vi "Lab Panel V4.87.vi"() -> ()   [LabVIEW 2013] (continued)
                        n2189 = case shown="True" w4030 {
                          tunnel: w4037 -> [_ w4069]
                          tunnel: w4036 -> [_ w4076]
                          tunnel: w4035 -> [_ _]
                          tunnel: w4034 -> [_ _]
                          tunnel: w4033 -> [_ w4075]
                          tunnel: w4032 -> [_ w4074]
                          tunnel: w4031 -> [_ w4039]
                          tunnel: w4028 -> [_ w4071]
                          tunnel: w4027 -> [_ w4070]
                          tunnel: w4026 -> [_ w4068]
                          tunnel: w4025 -> [_ w4060]
                          frame False {
                          }
                          frame True {
                            n2190 = local read "TDMS LAB03-1"() -> (w4073:refnum<k34>)
                            n2191 = Build Array(w4070) -> (w4065:dbl[])
                            n2192 = Build Array(w4068) -> (w4064:dbl[])
                            n2193 = Build Array(w4075) -> (w4063:dbl[])
                            n2194 = Build Array(w4076) -> (w4062:dbl[])
                            n2195 = Build Array(w4071) -> (w4067:dbl[])
                            n2196 = Build Array(w4069) -> (w4066:dbl[])
                            n2197 = Build Array(w4074) -> (w4061:dbl[])
                            n2198 = Build Array("AMPS ON", "AMPS OFF", "VOLTS", "PF", "TEMP Live", "TEMP Neut", "CYCLE") -> (w4044:string[])
                            n2199 = Bundle By Name("Y"=w4067, "t0"=w4060) -> (w4059:waveform(dbl))  [unwired: 1 in]
                            n2200 = Bundle By Name("Y"=w4066, "t0"=w4060) -> (w4058:waveform(dbl))  [unwired: 1 in]
                            n2201 = Bundle By Name("Y"=w4065, "t0"=w4060) -> (w4057:waveform(dbl))  [unwired: 1 in]
                            n2202 = Bundle By Name("Y"=w4064, "t0"=w4060) -> (w4056:waveform(dbl))  [unwired: 1 in]
                            n2203 = Bundle By Name("Y"=w4063, "t0"=w4060) -> (w4055:waveform(dbl))  [unwired: 1 in]
                            n2204 = Bundle By Name("Y"=w4062, "t0"=w4060) -> (w4054:waveform(dbl))  [unwired: 1 in]
                            n2205 = Bundle By Name("Y"=w4061, "t0"=w4060) -> (w4053:waveform(dbl))  [unwired: 1 in]
                            n2206 = Build Array(w4059, w4058, w4057, w4056, w4055, w4054, w4053) -> (w4052:waveform(dbl)[])
                            n2207 = TDMS Write(0:w4073, 5:"TEST VALUES", 7:w4044, 9:w4052) -> (4:w4043:refnum<k34>, 6:w4042:string, 15:w4041:errorcluster)  [unwired: 2 in, 1 out]
                            n2208 = TDMS Write(0:w4043, 5:w4042, 7:"TIME", 9:w4039, 11:w4041) -> (15:w4038:errorcluster)  [unwired: 1 in, 3 out]
                            n2209 = local write "data file error"(w4038) -> ()
                          }
                        }
                      }
                    }
                  }
                }
              }
              frame #5 {
                n2210 = case shown="True" w4077 {
                  tunnel: w4081 -> [_ w4086]
                  tunnel: w4080 -> [_ w4085]
                  tunnel: w4079 -> [_ w4083]
                  tunnel: w4078 -> [_ w4082]
                  frame False {
                  }
                  frame True {
                    n2211 = local read "DISP LAB03-2"() -> (w4087:T4)
                    n2212 = local read "SIG LAB03-2"() -> (w4088:T2)
                    n2213 = local read "ON L03-2"() -> (w4084:cluster{"amps":dbl, "volts":dbl, "pf":dbl})
                    n2214 = Unbundle(w4088) -> ("AMPS"=w4094:dbl, "VOLTS"=w4092:dbl, "PF"=w4091:dbl, "Tmp Live"=w4090:dbl, "Tmp Neut"=w4093:dbl)
                    n2215 = Unbundle(w4087) -> ("CYCLE"=w4089:dbl)  [unwired: 2 out]
                    n2216 = stacked-sequence {
                      tunnel: w4094 -> [w4098 w4117]
                      tunnel: w4093 -> [_ w4116]
                      tunnel: w4092 -> [w4097 w4115]
                      tunnel: w4091 -> [w4096 w4114]
                      tunnel: w4090 -> [_ w4113]
                      tunnel: w4089 -> [_ w4112]
                      tunnel: w4086 -> [_ w4111]
                      tunnel: w4085 -> [w4099 _]
                      tunnel: w4084 -> [w4095 w4109]
                      tunnel: w4083 -> [_ w4110]
                      tunnel: w4082 -> [_ w4105]
                      frame #0 {
                        n2217 = case shown="True" w4099 {
                          tunnel: w4098 -> [_ w4104]
                          tunnel: w4097 -> [_ w4103]
                          tunnel: w4096 -> [_ w4102]
                          tunnel: w4095 -> [_ w4100]
                          frame False {
                          }
                          frame True {
                            n2218 = Bundle(cluster=w4100, "amps"=w4104, "volts"=w4103, "pf"=w4102) -> (w4101:cluster{"amps":dbl, "volts":dbl, "pf":dbl})
                            n2219 = local write "ON L03-2"(w4101) -> ()
                          }
                        }
                      }
                      frame #1 {
                        n2220 = Unbundle(w4109) -> ("amps"=w4108:dbl, "volts"=w4107:dbl, "pf"=w4106:dbl)
                        n2221 = case shown="True" w4110 {
                          tunnel: w4117 -> [_ w4149]
                          tunnel: w4116 -> [_ w4156]
                          tunnel: w4115 -> [_ _]
                          tunnel: w4114 -> [_ _]
                          tunnel: w4113 -> [_ w4155]
                          tunnel: w4112 -> [_ w4154]
                          tunnel: w4111 -> [_ w4119]
                          tunnel: w4108 -> [_ w4151]
                          tunnel: w4107 -> [_ w4150]
                          tunnel: w4106 -> [_ w4148]
                          tunnel: w4105 -> [_ w4140]
                          frame False {
                          }
                          frame True {
                            n2222 = local read "TDMS LAB03-2"() -> (w4153:refnum<k34>)
                            n2223 = Build Array(w4150) -> (w4145:dbl[])
                            n2224 = Build Array(w4148) -> (w4144:dbl[])
                            n2225 = Build Array(w4155) -> (w4143:dbl[])
                            n2226 = Build Array(w4156) -> (w4142:dbl[])
                            n2227 = Build Array(w4151) -> (w4147:dbl[])
                            n2228 = Build Array(w4149) -> (w4146:dbl[])
                            n2229 = Build Array(w4154) -> (w4141:dbl[])
                            n2230 = Build Array("AMPS ON", "AMPS OFF", "VOLTS", "PF", "TEMP Live", "TEMP Neut", "CYCLE") -> (w4124:string[])
                            n2231 = Bundle By Name("Y"=w4147, "t0"=w4140) -> (w4139:waveform(dbl))  [unwired: 1 in]
                            n2232 = Bundle By Name("Y"=w4146, "t0"=w4140) -> (w4138:waveform(dbl))  [unwired: 1 in]
                            n2233 = Bundle By Name("Y"=w4145, "t0"=w4140) -> (w4137:waveform(dbl))  [unwired: 1 in]
                            n2234 = Bundle By Name("Y"=w4144, "t0"=w4140) -> (w4136:waveform(dbl))  [unwired: 1 in]
                            n2235 = Bundle By Name("Y"=w4143, "t0"=w4140) -> (w4135:waveform(dbl))  [unwired: 1 in]
                            n2236 = Bundle By Name("Y"=w4142, "t0"=w4140) -> (w4134:waveform(dbl))  [unwired: 1 in]
                            n2237 = Bundle By Name("Y"=w4141, "t0"=w4140) -> (w4133:waveform(dbl))  [unwired: 1 in]
                            n2238 = Build Array(w4139, w4138, w4137, w4136, w4135, w4134, w4133) -> (w4132:waveform(dbl)[])
                            n2239 = TDMS Write(0:w4153, 5:"TEST VALUES", 7:w4124, 9:w4132) -> (4:w4123:refnum<k34>, 6:w4122:string, 15:w4121:errorcluster)  [unwired: 2 in, 1 out]
                            n2240 = TDMS Write(0:w4123, 5:w4122, 7:"TIME", 9:w4119, 11:w4121) -> (15:w4118:errorcluster)  [unwired: 1 in, 3 out]
                            n2241 = local write "data file error"(w4118) -> ()
                          }
                        }
                      }
                    }
                  }
                }
              }
              frame #6 {
                n2242 = case shown="True" w4157 {
                  tunnel: w4161 -> [_ w4166]
                  tunnel: w4160 -> [_ w4165]
                  tunnel: w4159 -> [_ w4163]
                  tunnel: w4158 -> [_ w4162]
                  frame False {
                  }
                  frame True {
                    n2243 = local read "DISP LAB04-1"() -> (w4167:T4)
                    n2244 = local read "SIG LAB04-1"() -> (w4168:T2)
                    n2245 = local read "ON L04-1"() -> (w4164:cluster{"amps":dbl, "volts":dbl, "pf":dbl})
                    n2246 = Unbundle(w4168) -> ("AMPS"=w4174:dbl, "VOLTS"=w4172:dbl, "PF"=w4171:dbl, "Tmp Live"=w4170:dbl, "Tmp Neut"=w4173:dbl)
                    n2247 = Unbundle(w4167) -> ("CYCLE"=w4169:dbl)  [unwired: 2 out]
                    n2248 = stacked-sequence {
                      tunnel: w4174 -> [w4178 w4197]
                      tunnel: w4173 -> [_ w4196]
                      tunnel: w4172 -> [w4177 w4195]
                      tunnel: w4171 -> [w4176 w4194]
                      tunnel: w4170 -> [_ w4193]
                      tunnel: w4169 -> [_ w4192]
                      tunnel: w4166 -> [_ w4191]
                      tunnel: w4165 -> [w4179 _]
                      tunnel: w4164 -> [w4175 w4189]
                      tunnel: w4163 -> [_ w4190]
                      tunnel: w4162 -> [_ w4185]
                      frame #0 {
                        n2249 = case shown="True" w4179 {
                          tunnel: w4178 -> [_ w4184]
                          tunnel: w4177 -> [_ w4183]
                          tunnel: w4176 -> [_ w4182]
                          tunnel: w4175 -> [_ w4180]
                          frame False {
                          }
                          frame True {
                            n2250 = Bundle(cluster=w4180, "amps"=w4184, "volts"=w4183, "pf"=w4182) -> (w4181:cluster{"amps":dbl, "volts":dbl, "pf":dbl})
                            n2251 = local write "ON L04-1"(w4181) -> ()
                          }
                        }
                      }
                      frame #1 {
                        n2252 = Unbundle(w4189) -> ("amps"=w4188:dbl, "volts"=w4187:dbl, "pf"=w4186:dbl)
                        n2253 = case shown="True" w4190 {
                          tunnel: w4197 -> [_ w4229]
                          tunnel: w4196 -> [_ w4236]
                          tunnel: w4195 -> [_ _]
                          tunnel: w4194 -> [_ _]
                          tunnel: w4193 -> [_ w4235]
                          tunnel: w4192 -> [_ w4234]
                          tunnel: w4191 -> [_ w4199]
                          tunnel: w4188 -> [_ w4231]
                          tunnel: w4187 -> [_ w4230]
                          tunnel: w4186 -> [_ w4228]
                          tunnel: w4185 -> [_ w4220]
                          frame False {
                          }
                          frame True {
                            n2254 = local read "TDMS LAB04-1"() -> (w4233:refnum<k34>)
                            n2255 = Build Array(w4230) -> (w4225:dbl[])
                            n2256 = Build Array(w4228) -> (w4224:dbl[])
                            n2257 = Build Array(w4235) -> (w4223:dbl[])
                            n2258 = Build Array(w4236) -> (w4222:dbl[])
                            n2259 = Build Array(w4231) -> (w4227:dbl[])
                            n2260 = Build Array(w4229) -> (w4226:dbl[])
                            n2261 = Build Array(w4234) -> (w4221:dbl[])
                            n2262 = Build Array("AMPS ON", "AMPS OFF", "VOLTS", "PF", "TEMP Live", "TEMP Neut", "CYCLE") -> (w4204:string[])
                            n2263 = Bundle By Name("Y"=w4227, "t0"=w4220) -> (w4219:waveform(dbl))  [unwired: 1 in]
                            n2264 = Bundle By Name("Y"=w4226, "t0"=w4220) -> (w4218:waveform(dbl))  [unwired: 1 in]
                            n2265 = Bundle By Name("Y"=w4225, "t0"=w4220) -> (w4217:waveform(dbl))  [unwired: 1 in]
                            n2266 = Bundle By Name("Y"=w4224, "t0"=w4220) -> (w4216:waveform(dbl))  [unwired: 1 in]
                            n2267 = Bundle By Name("Y"=w4223, "t0"=w4220) -> (w4215:waveform(dbl))  [unwired: 1 in]
                            n2268 = Bundle By Name("Y"=w4222, "t0"=w4220) -> (w4214:waveform(dbl))  [unwired: 1 in]
                            n2269 = Bundle By Name("Y"=w4221, "t0"=w4220) -> (w4213:waveform(dbl))  [unwired: 1 in]
                            n2270 = Build Array(w4219, w4218, w4217, w4216, w4215, w4214, w4213) -> (w4212:waveform(dbl)[])
                            n2271 = TDMS Write(0:w4233, 5:"TEST VALUES", 7:w4204, 9:w4212) -> (4:w4203:refnum<k34>, 6:w4202:string, 15:w4201:errorcluster)  [unwired: 2 in, 1 out]
                            n2272 = TDMS Write(0:w4203, 5:w4202, 7:"TIME", 9:w4199, 11:w4201) -> (15:w4198:errorcluster)  [unwired: 1 in, 3 out]
                            n2273 = local write "data file error"(w4198) -> ()
                          }
                        }
                      }
                    }
                  }
                }
              }
              frame #7 {
                n2274 = case shown="True" w4237 {
                  tunnel: w4241 -> [_ w4246]
                  tunnel: w4240 -> [_ w4245]
                  tunnel: w4239 -> [_ w4243]
                  tunnel: w4238 -> [_ w4242]
                  frame False {
                  }
                  frame True {
                    n2275 = local read "DISP LAB04-2"() -> (w4247:T4)
                    n2276 = local read "SIG LAB04-2"() -> (w4248:T2)
                    n2277 = local read "ON L04-2"() -> (w4244:cluster{"amps":dbl, "volts":dbl, "pf":dbl})
                    n2278 = Unbundle(w4248) -> ("AMPS"=w4254:dbl, "VOLTS"=w4252:dbl, "PF"=w4251:dbl, "Tmp Live"=w4250:dbl, "Tmp Neut"=w4253:dbl)
                    n2279 = Unbundle(w4247) -> ("CYCLE"=w4249:dbl)  [unwired: 2 out]
                    n2280 = stacked-sequence {
                      tunnel: w4254 -> [w4258 w4277]
                      tunnel: w4253 -> [_ w4276]
                      tunnel: w4252 -> [w4257 w4275]
                      tunnel: w4251 -> [w4256 w4274]
                      tunnel: w4250 -> [_ w4273]
                      tunnel: w4249 -> [_ w4272]
                      tunnel: w4246 -> [_ w4271]
                      tunnel: w4245 -> [w4259 _]
                      tunnel: w4244 -> [w4255 w4269]
                      tunnel: w4243 -> [_ w4270]
                      tunnel: w4242 -> [_ w4265]
                      frame #0 {
                        n2281 = case shown="True" w4259 {
                          tunnel: w4258 -> [_ w4264]
                          tunnel: w4257 -> [_ w4263]
                          tunnel: w4256 -> [_ w4262]
                          tunnel: w4255 -> [_ w4260]
                          frame False {
                          }
                          frame True {
                            n2282 = Bundle(cluster=w4260, "amps"=w4264, "volts"=w4263, "pf"=w4262) -> (w4261:cluster{"amps":dbl, "volts":dbl, "pf":dbl})
                            n2283 = local write "ON L04-2"(w4261) -> ()
                          }
                        }
                      }
                      frame #1 {
                        n2284 = Unbundle(w4269) -> ("amps"=w4268:dbl, "volts"=w4267:dbl, "pf"=w4266:dbl)
                        n2285 = case shown="True" w4270 {
                          tunnel: w4277 -> [_ w4309]
                          tunnel: w4276 -> [_ w4316]
                          tunnel: w4275 -> [_ _]
                          tunnel: w4274 -> [_ _]
                          tunnel: w4273 -> [_ w4315]
                          tunnel: w4272 -> [_ w4314]
                          tunnel: w4271 -> [_ w4279]
                          tunnel: w4268 -> [_ w4311]
                          tunnel: w4267 -> [_ w4310]
                          tunnel: w4266 -> [_ w4308]
                          tunnel: w4265 -> [_ w4300]
                          frame False {
                          }
                          frame True {
                            n2286 = local read "TDMS LAB04-2"() -> (w4313:refnum<k34>)
                            n2287 = Build Array(w4310) -> (w4305:dbl[])
                            n2288 = Build Array(w4308) -> (w4304:dbl[])
                            n2289 = Build Array(w4315) -> (w4303:dbl[])
                            n2290 = Build Array(w4316) -> (w4302:dbl[])
                            n2291 = Build Array(w4311) -> (w4307:dbl[])
                            n2292 = Build Array(w4309) -> (w4306:dbl[])
                            n2293 = Build Array(w4314) -> (w4301:dbl[])
                            n2294 = Build Array("AMPS ON", "AMPS OFF", "VOLTS", "PF", "TEMP Live", "TEMP Neut", "CYCLE") -> (w4284:string[])
                            n2295 = Bundle By Name("Y"=w4307, "t0"=w4300) -> (w4299:waveform(dbl))  [unwired: 1 in]
                            n2296 = Bundle By Name("Y"=w4306, "t0"=w4300) -> (w4298:waveform(dbl))  [unwired: 1 in]
                            n2297 = Bundle By Name("Y"=w4305, "t0"=w4300) -> (w4297:waveform(dbl))  [unwired: 1 in]
                            n2298 = Bundle By Name("Y"=w4304, "t0"=w4300) -> (w4296:waveform(dbl))  [unwired: 1 in]
                            n2299 = Bundle By Name("Y"=w4303, "t0"=w4300) -> (w4295:waveform(dbl))  [unwired: 1 in]
                            n2300 = Bundle By Name("Y"=w4302, "t0"=w4300) -> (w4294:waveform(dbl))  [unwired: 1 in]
                            n2301 = Bundle By Name("Y"=w4301, "t0"=w4300) -> (w4293:waveform(dbl))  [unwired: 1 in]
                            n2302 = Build Array(w4299, w4298, w4297, w4296, w4295, w4294, w4293) -> (w4292:waveform(dbl)[])
                            n2303 = TDMS Write(0:w4313, 5:"TEST VALUES", 7:w4284, 9:w4292) -> (4:w4283:refnum<k34>, 6:w4282:string, 15:w4281:errorcluster)  [unwired: 2 in, 1 out]
                            n2304 = TDMS Write(0:w4283, 5:w4282, 7:"TIME", 9:w4279, 11:w4281) -> (15:w4278:errorcluster)  [unwired: 1 in, 3 out]
                            n2305 = local write "data file error"(w4278) -> ()
                          }
                        }
                      }
                    }
                  }
                }
              }
              frame #8 {
                n2306 = case shown="True" w4317 {
                  tunnel: w4321 -> [_ w4326]
                  tunnel: w4320 -> [_ w4325]
                  tunnel: w4319 -> [_ w4323]
                  tunnel: w4318 -> [_ w4322]
                  frame False {
                  }
                  frame True {
                    n2307 = local read "DISP LAB05-1"() -> (w4327:T4)
                    n2308 = local read "SIG LAB05-1"() -> (w4328:T2)
                    n2309 = local read "ON L05-1"() -> (w4324:cluster{"amps":dbl, "volts":dbl, "pf":dbl})
                    n2310 = Unbundle(w4328) -> ("AMPS"=w4334:dbl, "VOLTS"=w4332:dbl, "PF"=w4331:dbl, "Tmp Live"=w4330:dbl, "Tmp Neut"=w4333:dbl)
                    n2311 = Unbundle(w4327) -> ("CYCLE"=w4329:dbl)  [unwired: 2 out]
                    n2312 = stacked-sequence {
                      tunnel: w4334 -> [w4338 w4357]
                      tunnel: w4333 -> [_ w4356]
                      tunnel: w4332 -> [w4337 w4355]
                      tunnel: w4331 -> [w4336 w4354]
                      tunnel: w4330 -> [_ w4353]
                      tunnel: w4329 -> [_ w4352]
                      tunnel: w4326 -> [_ w4351]
                      tunnel: w4325 -> [w4339 _]
                      tunnel: w4324 -> [w4335 w4349]
                      tunnel: w4323 -> [_ w4350]
                      tunnel: w4322 -> [_ w4345]
                      frame #0 {
                        n2313 = case shown="True" w4339 {
                          tunnel: w4338 -> [_ w4344]
                          tunnel: w4337 -> [_ w4343]
                          tunnel: w4336 -> [_ w4342]
                          tunnel: w4335 -> [_ w4340]
                          frame False {
                          }
                          frame True {
                            n2314 = Bundle(cluster=w4340, "amps"=w4344, "volts"=w4343, "pf"=w4342) -> (w4341:cluster{"amps":dbl, "volts":dbl, "pf":dbl})
                            n2315 = local write "ON L05-1"(w4341) -> ()
                          }
                        }
                      }
                      frame #1 {
                        n2316 = Unbundle(w4349) -> ("amps"=w4348:dbl, "volts"=w4347:dbl, "pf"=w4346:dbl)
                        n2317 = case shown="True" w4350 {
                          tunnel: w4357 -> [_ w4389]
                          tunnel: w4356 -> [_ w4396]
                          tunnel: w4355 -> [_ _]
                          tunnel: w4354 -> [_ _]
                          tunnel: w4353 -> [_ w4395]
                          tunnel: w4352 -> [_ w4394]
                          tunnel: w4351 -> [_ w4359]
                          tunnel: w4348 -> [_ w4391]
                          tunnel: w4347 -> [_ w4390]
                          tunnel: w4346 -> [_ w4388]
                          tunnel: w4345 -> [_ w4380]
                          frame False {
                          }
                          frame True {
                            n2318 = local read "TDMS LAB05-1"() -> (w4393:refnum<k34>)
                            n2319 = Build Array(w4390) -> (w4385:dbl[])
                            n2320 = Build Array(w4388) -> (w4384:dbl[])
                            n2321 = Build Array(w4395) -> (w4383:dbl[])
                            n2322 = Build Array(w4396) -> (w4382:dbl[])
                            n2323 = Build Array(w4391) -> (w4387:dbl[])
                            n2324 = Build Array(w4389) -> (w4386:dbl[])
                            n2325 = Build Array(w4394) -> (w4381:dbl[])
                            n2326 = Build Array("AMPS ON", "AMPS OFF", "VOLTS", "PF", "TEMP Live", "TEMP Neut", "CYCLE") -> (w4364:string[])
                            n2327 = Bundle By Name("Y"=w4387, "t0"=w4380) -> (w4379:waveform(dbl))  [unwired: 1 in]
                            n2328 = Bundle By Name("Y"=w4386, "t0"=w4380) -> (w4378:waveform(dbl))  [unwired: 1 in]
                            n2329 = Bundle By Name("Y"=w4385, "t0"=w4380) -> (w4377:waveform(dbl))  [unwired: 1 in]
                            n2330 = Bundle By Name("Y"=w4384, "t0"=w4380) -> (w4376:waveform(dbl))  [unwired: 1 in]
                            n2331 = Bundle By Name("Y"=w4383, "t0"=w4380) -> (w4375:waveform(dbl))  [unwired: 1 in]
                            n2332 = Bundle By Name("Y"=w4382, "t0"=w4380) -> (w4374:waveform(dbl))  [unwired: 1 in]
                            n2333 = Bundle By Name("Y"=w4381, "t0"=w4380) -> (w4373:waveform(dbl))  [unwired: 1 in]
                            n2334 = Build Array(w4379, w4378, w4377, w4376, w4375, w4374, w4373) -> (w4372:waveform(dbl)[])
                            n2335 = TDMS Write(0:w4393, 5:"TEST VALUES", 7:w4364, 9:w4372) -> (4:w4363:refnum<k34>, 6:w4362:string, 15:w4361:errorcluster)  [unwired: 2 in, 1 out]
                            n2336 = TDMS Write(0:w4363, 5:w4362, 7:"TIME", 9:w4359, 11:w4361) -> (15:w4358:errorcluster)  [unwired: 1 in, 3 out]
                            n2337 = local write "data file error"(w4358) -> ()
                          }
                        }
                      }
                    }
                  }
                }
              }
              frame #9 {
                n2338 = case shown="True" w4397 {
                  tunnel: w4401 -> [_ w4406]
                  tunnel: w4400 -> [_ w4405]
                  tunnel: w4399 -> [_ w4403]
                  tunnel: w4398 -> [_ w4402]
                  frame False {
                  }
                  frame True {
                    n2339 = local read "DISP LAB05-2"() -> (w4407:T4)
                    n2340 = local read "SIG LAB05-2"() -> (w4408:T2)
                    n2341 = local read "ON L05-2"() -> (w4404:cluster{"amps":dbl, "volts":dbl, "pf":dbl})
                    n2342 = Unbundle(w4408) -> ("AMPS"=w4414:dbl, "VOLTS"=w4412:dbl, "PF"=w4411:dbl, "Tmp Live"=w4410:dbl, "Tmp Neut"=w4413:dbl)
                    n2343 = Unbundle(w4407) -> ("CYCLE"=w4409:dbl)  [unwired: 2 out]
                    n2344 = stacked-sequence {
                      tunnel: w4414 -> [w4418 w4437]
                      tunnel: w4413 -> [_ w4436]
                      tunnel: w4412 -> [w4417 w4435]
                      tunnel: w4411 -> [w4416 w4434]
                      tunnel: w4410 -> [_ w4433]
                      tunnel: w4409 -> [_ w4432]
                      tunnel: w4406 -> [_ w4431]
                      tunnel: w4405 -> [w4419 _]
                      tunnel: w4404 -> [w4415 w4429]
                      tunnel: w4403 -> [_ w4430]
                      tunnel: w4402 -> [_ w4425]
                      frame #0 {
                        n2345 = case shown="True" w4419 {
                          tunnel: w4418 -> [_ w4424]
                          tunnel: w4417 -> [_ w4423]
                          tunnel: w4416 -> [_ w4422]
                          tunnel: w4415 -> [_ w4420]
                          frame False {
                          }
                          frame True {
                            n2346 = Bundle(cluster=w4420, "amps"=w4424, "volts"=w4423, "pf"=w4422) -> (w4421:cluster{"amps":dbl, "volts":dbl, "pf":dbl})
                            n2347 = local write "ON L05-2"(w4421) -> ()
                          }
                        }
                      }
                      frame #1 {
                        n2348 = Unbundle(w4429) -> ("amps"=w4428:dbl, "volts"=w4427:dbl, "pf"=w4426:dbl)
                        n2349 = case shown="True" w4430 {
                          tunnel: w4437 -> [_ w4469]
                          tunnel: w4436 -> [_ w4476]
                          tunnel: w4435 -> [_ _]
                          tunnel: w4434 -> [_ _]
                          tunnel: w4433 -> [_ w4475]
                          tunnel: w4432 -> [_ w4474]
                          tunnel: w4431 -> [_ w4439]
                          tunnel: w4428 -> [_ w4471]
                          tunnel: w4427 -> [_ w4470]
                          tunnel: w4426 -> [_ w4468]
                          tunnel: w4425 -> [_ w4460]
                          frame False {
                          }
                          frame True {
                            n2350 = local read "TDMS LAB05-2"() -> (w4473:refnum<k34>)
                            n2351 = Build Array(w4470) -> (w4465:dbl[])
                            n2352 = Build Array(w4468) -> (w4464:dbl[])
                            n2353 = Build Array(w4475) -> (w4463:dbl[])
                            n2354 = Build Array(w4476) -> (w4462:dbl[])
                            n2355 = Build Array(w4471) -> (w4467:dbl[])
                            n2356 = Build Array(w4469) -> (w4466:dbl[])
                            n2357 = Build Array(w4474) -> (w4461:dbl[])
                            n2358 = Build Array("AMPS ON", "AMPS OFF", "VOLTS", "PF", "TEMP Live", "TEMP Neut", "CYCLE") -> (w4444:string[])
                            n2359 = Bundle By Name("Y"=w4467, "t0"=w4460) -> (w4459:waveform(dbl))  [unwired: 1 in]
                            n2360 = Bundle By Name("Y"=w4466, "t0"=w4460) -> (w4458:waveform(dbl))  [unwired: 1 in]
                            n2361 = Bundle By Name("Y"=w4465, "t0"=w4460) -> (w4457:waveform(dbl))  [unwired: 1 in]
                            n2362 = Bundle By Name("Y"=w4464, "t0"=w4460) -> (w4456:waveform(dbl))  [unwired: 1 in]
                            n2363 = Bundle By Name("Y"=w4463, "t0"=w4460) -> (w4455:waveform(dbl))  [unwired: 1 in]
                            n2364 = Bundle By Name("Y"=w4462, "t0"=w4460) -> (w4454:waveform(dbl))  [unwired: 1 in]
                            n2365 = Bundle By Name("Y"=w4461, "t0"=w4460) -> (w4453:waveform(dbl))  [unwired: 1 in]
                            n2366 = Build Array(w4459, w4458, w4457, w4456, w4455, w4454, w4453) -> (w4452:waveform(dbl)[])
                            n2367 = TDMS Write(0:w4473, 5:"TEST VALUES", 7:w4444, 9:w4452) -> (4:w4443:refnum<k34>, 6:w4442:string, 15:w4441:errorcluster)  [unwired: 2 in, 1 out]
                            n2368 = TDMS Write(0:w4443, 5:w4442, 7:"TIME", 9:w4439, 11:w4441) -> (15:w4438:errorcluster)  [unwired: 1 in, 3 out]
                            n2369 = local write "data file error"(w4438) -> ()
                          }
                        }
                      }
                    }
                  }
                }
              }
            }
          }
          frame #13 {
            # "display test values on chart"
            n2370 = local read "jig cycle"() -> (w4481:dbl)
            n2371 = local read "on loops"() -> (w4483:dbl)
            n2372 = Add(x=w4483, y=2) -> (x+y=w4480:dbl)
            n2373 = Equal?(x=w4481, y=1) -> (x = y?=w4479:bool)
            n2374 = Equal?(x=w4481, y=w4480) -> (x = y?=w4478:bool)
            n2375 = Or(x=w4479, y=w4478) -> (x .or. y?=w4477:bool)
            "graph flag" <- w4477
            n2376 = global write "Global display 3.vi" "graph flag"(w4477) -> ()
            n2377 = case shown="True" w4477 {
              frame False {
              }
              frame True {
                n2378 = local read "SIG LAB05-1"() -> (w4526:T2)
                n2379 = local read "SIG LAB04-2"() -> (w4527:T2)
                n2380 = local read "SIG LAB05-2"() -> (w4525:T2)
                n2381 = local read "SIG LAB04-1"() -> (w4528:T2)
                n2382 = local read "SIG LAB03-1"() -> (w4530:T2)
                n2383 = local read "SIG LAB03-2"() -> (w4529:T2)
                n2384 = local read "SIG LAB01-1"() -> (w4534:T2)
                n2385 = local read "SIG LAB02-2"() -> (w4531:T2)
                n2386 = local read "SIG LAB02-1"() -> (w4532:T2)
                n2387 = local read "SIG LAB01-2"() -> (w4533:T2)
                n2388 = Unbundle(w4527) -> ("AMPS"=w4517:dbl, "VOLTS"=w4507:dbl, "Tmp Live"=w4497:dbl, "Tmp Neut"=w4487:dbl)  [unwired: 1 out]
                n2389 = Unbundle(w4526) -> ("AMPS"=w4516:dbl, "VOLTS"=w4506:dbl, "Tmp Live"=w4496:dbl, "Tmp Neut"=w4486:dbl)  [unwired: 1 out]
                n2390 = Unbundle(w4525) -> ("AMPS"=w4515:dbl, "VOLTS"=w4505:dbl, "Tmp Live"=w4495:dbl, "Tmp Neut"=w4485:dbl)  [unwired: 1 out]
                n2391 = Unbundle(w4528) -> ("AMPS"=w4518:dbl, "VOLTS"=w4508:dbl, "Tmp Live"=w4498:dbl, "Tmp Neut"=w4488:dbl)  [unwired: 1 out]
                n2392 = Unbundle(w4529) -> ("AMPS"=w4519:dbl, "VOLTS"=w4509:dbl, "Tmp Live"=w4499:dbl, "Tmp Neut"=w4489:dbl)  [unwired: 1 out]
                n2393 = Unbundle(w4530) -> ("AMPS"=w4520:dbl, "VOLTS"=w4510:dbl, "Tmp Live"=w4500:dbl, "Tmp Neut"=w4490:dbl)  [unwired: 1 out]
                n2394 = Unbundle(w4531) -> ("AMPS"=w4521:dbl, "VOLTS"=w4511:dbl, "Tmp Live"=w4501:dbl, "Tmp Neut"=w4491:dbl)  [unwired: 1 out]
                n2395 = Unbundle(w4532) -> ("AMPS"=w4522:dbl, "VOLTS"=w4512:dbl, "Tmp Live"=w4502:dbl, "Tmp Neut"=w4492:dbl)  [unwired: 1 out]
                n2396 = Unbundle(w4534) -> ("AMPS"=w4524:dbl, "VOLTS"=w4514:dbl, "Tmp Live"=w4504:dbl, "Tmp Neut"=w4494:dbl)  [unwired: 1 out]
                n2397 = Unbundle(w4533) -> ("AMPS"=w4523:dbl, "VOLTS"=w4513:dbl, "Tmp Live"=w4503:dbl, "Tmp Neut"=w4493:dbl)  [unwired: 1 out]
                n2398 = stacked-sequence {
                  tunnel: w4524 -> [w4566 _ _]
                  tunnel: w4523 -> [w4565 _ _]
                  tunnel: w4522 -> [w4556 _ _]
                  tunnel: w4521 -> [w4555 _ _]
                  tunnel: w4520 -> [w4545 _ _]
                  tunnel: w4519 -> [w4544 _ _]
                  tunnel: w4518 -> [_ w4589 _]
                  tunnel: w4517 -> [_ w4588 _]
                  tunnel: w4516 -> [_ w4578 _]
                  tunnel: w4515 -> [_ w4577 _]
                  tunnel: w4514 -> [w4563 _ _]
                  tunnel: w4513 -> [w4562 _ _]
                  tunnel: w4512 -> [w4553 _ _]
                  tunnel: w4511 -> [w4552 _ _]
                  tunnel: w4510 -> [w4543 _ _]
                  tunnel: w4509 -> [w4542 _ _]
                  tunnel: w4508 -> [_ w4587 _]
                  tunnel: w4507 -> [_ w4586 _]
                  tunnel: w4506 -> [_ w4576 _]
                  tunnel: w4505 -> [_ w4575 _]
                  tunnel: w4504 -> [w4560 _ _]
                  tunnel: w4503 -> [w4558 _ _]
                  tunnel: w4502 -> [w4549 _ _]
                  tunnel: w4501 -> [w4547 _ _]
                  tunnel: w4500 -> [w4541 _ _]
                  tunnel: w4499 -> [w4539 _ _]
                  tunnel: w4498 -> [_ w4585 _]
                  tunnel: w4497 -> [_ w4583 _]
                  tunnel: w4496 -> [_ w4574 _]
                  tunnel: w4495 -> [_ w4572 _]
                  tunnel: w4494 -> [w4559 _ _]
                  tunnel: w4493 -> [w4557 _ _]
                  tunnel: w4492 -> [w4548 _ _]
                  tunnel: w4491 -> [w4546 _ _]
                  tunnel: w4490 -> [w4540 _ _]
                  tunnel: w4489 -> [w4538 _ _]
                  tunnel: w4488 -> [_ w4584 _]
                  tunnel: w4487 -> [_ w4582 _]
                  tunnel: w4486 -> [_ w4573 _]
                  tunnel: w4485 -> [_ w4571 _]
                  frame #0 {
                    n2399 = Merge Signals(w4566, w4565) -> (→"LAB01 AMPS":dynamicdata)
                    n2400 = Merge Signals(w4563, w4562) -> (→"LAB01 VOLTS":dynamicdata)
                    n2401 = Merge Signals(w4543, w4542) -> (→"LAB03 VOLTS":dynamicdata)
                    n2402 = Merge Signals(w4560, w4559, w4558, w4557) -> (→"LAB01 deg C":dynamicdata)
                    n2403 = Merge Signals(w4556, w4555) -> (→"LAB02 AMPS":dynamicdata)
                    n2404 = Merge Signals(w4549, w4548, w4547, w4546) -> (→"LAB02 deg C":dynamicdata)
                    n2405 = Merge Signals(w4541, w4540, w4539, w4538) -> (→"LAB03 deg C":dynamicdata)
                    n2406 = Merge Signals(w4553, w4552) -> (→"LAB02 VOLTS":dynamicdata)
                    n2407 = Merge Signals(w4545, w4544) -> (→"LAB03 AMPS":dynamicdata)
                  }
                  frame #1 {
                    n2408 = Merge Signals(w4576, w4575) -> (→"LAB05 VOLTS":dynamicdata)
                    n2409 = Merge Signals(w4589, w4588) -> (→"LAB04 AMPS":dynamicdata)
                    n2410 = Merge Signals(w4578, w4577) -> (→"LAB05 AMPS":dynamicdata)
                    n2411 = Merge Signals(w4574, w4573, w4572, w4571) -> (→"LAB05 deg C":dynamicdata)
                    n2412 = Merge Signals(w4585, w4584, w4583, w4582) -> (→"LAB04 deg C":dynamicdata)
                    n2413 = Merge Signals(w4587, w4586) -> (→"LAB04 VOLTS":dynamicdata)
                  }
                  frame #2 {
                    n2414 = local read "LAB05 VOLTS"() -> (w4597:dynamicdata)
                    n2415 = local read "LAB04 VOLTS"() -> (w4598:dynamicdata)
                    n2416 = local read "LAB02 VOLTS"() -> (w4600:dynamicdata)
                    n2417 = local read "LAB03 VOLTS"() -> (w4599:dynamicdata)
                    n2418 = local read "LAB05 AMPS"() -> (w4603:dynamicdata)
                    n2419 = local read "LAB01 VOLTS"() -> (w4601:dynamicdata)
                    n2420 = local read "LAB04 AMPS"() -> (w4604:dynamicdata)
                    n2421 = local read "LAB03 AMPS"() -> (w4605:dynamicdata)
                    n2422 = local read "LAB03 deg C"() -> (w4593:dynamicdata)
                    n2423 = local read "LAB02 AMPS"() -> (w4606:dynamicdata)
                    n2424 = local read "LAB04 deg C"() -> (w4592:dynamicdata)
                    n2425 = local read "LAB05 deg C"() -> (w4591:dynamicdata)
                    n2426 = local read "LAB02 deg C"() -> (w4594:dynamicdata)
                    n2427 = local read "LAB01 deg C"() -> (w4595:dynamicdata)
                    n2428 = local read "LAB01 AMPS"() -> (w4607:dynamicdata)
                    n2429 = Merge Signals(w4595, w4594, w4593, w4592, w4591) -> (w4590:dynamicdata)
                    n2430 = Merge Signals(w4607, w4606, w4605, w4604, w4603) -> (w4602:dynamicdata)
                    n2431 = Merge Signals(w4601, w4600, w4599, w4598, w4597) -> (w4596:dynamicdata)
                    n2432 = global write "Global display 3.vi" "graph volts"(w4596) -> ()
                    n2433 = global write "Global display 3.vi" "graph deg C"(w4590) -> ()
                    n2434 = global write "Global display 3.vi" "graph amps"(w4602) -> ()
                  }
                }
              }
            }
          }
          frame #14 {
            # "check for amps fail"
            # "check for cycle test & temperature rise fail conditions"
            n2435 = local read "on loops"() -> (w4634:dbl)
            n2436 = local read "jig cycle"() -> (w4631:dbl)
            n2437 = local read "jig cycle"() -> (w4636:dbl)
            n2438 = Add(x=w4634, y=3.0) -> (x+y=w4632:dbl)
            n2439 = Equal?(x=w4631, y=w4632) -> (x = y?=w4627:bool)
            n2440 = local read "Fail Loops"() -> (w4608:dbl)
            n2441 = Equal?(x=w4636, y=1.0) -> (x = y?=w4629:bool)
            n2442 = global write "Global 1.vi" "fail count"(w4608) -> ()
            n2443 = stacked-sequence {
              tunnel: w4630 -> [w4639 _ _ _ _ _ _ _ _ _]
              tunnel: w4629 -> [w4640 w4660 w4680 w4700 w4720 w4740 w4760 w4780 w4800 w4820]
              tunnel: w4628 -> [w4637 _ _ _ _ _ _ _ _ _]
              tunnel: w4627 -> [w4638 w4659 w4679 w4699 w4719 w4739 w4759 w4779 w4799 w4819]
              tunnel: w4626 -> [_ w4658 _ _ _ _ _ _ _ _]
              tunnel: w4625 -> [_ w4657 _ _ _ _ _ _ _ _]
              tunnel: w4624 -> [_ _ w4678 _ _ _ _ _ _ _]
              tunnel: w4623 -> [_ _ w4677 _ _ _ _ _ _ _]
              tunnel: w4622 -> [_ _ _ w4698 _ _ _ _ _ _]
              tunnel: w4621 -> [_ _ _ w4697 _ _ _ _ _ _]
              tunnel: w4620 -> [_ _ _ _ w4718 _ _ _ _ _]
              tunnel: w4619 -> [_ _ _ _ w4717 _ _ _ _ _]
              tunnel: w4618 -> [_ _ _ _ _ w4738 _ _ _ _]
              tunnel: w4617 -> [_ _ _ _ _ w4737 _ _ _ _]
              tunnel: w4616 -> [_ _ _ _ _ _ w4758 _ _ _]
              tunnel: w4615 -> [_ _ _ _ _ _ w4757 _ _ _]
              tunnel: w4614 -> [_ _ _ _ _ _ _ w4778 _ _]
              tunnel: w4613 -> [_ _ _ _ _ _ _ w4777 _ _]
              tunnel: w4612 -> [_ _ _ _ _ _ _ _ w4798 _]
              tunnel: w4611 -> [_ _ _ _ _ _ _ _ w4797 _]
              tunnel: w4610 -> [_ _ _ _ _ _ _ _ _ w4818]
              tunnel: w4609 -> [_ _ _ _ _ _ _ _ _ w4817]
              frame #0 {
                # "LAB01-1"
                n2444 = case shown="True" w4637 {
                  tunnel: w4640 -> [_ w4653]
                  tunnel: w4639 -> [_ w4650]
                  tunnel: w4638 -> [_ w4649]
                  frame False {
                  }
                  frame True {
                    n2445 = local read "TEMP START LAB01-1"() -> (w4655:cluster{"TL":dbl, "TN":dbl})
                    n2446 = local read "RESULT LAB01-1"() -> (w4644:bool)
                    n2447 = local read "FAIL LAB01-1"() -> (w4647:cluster{"LO":dbl, "HI":dbl})
                    n2448 = local read "TDMS LAB01-1"() -> (w4654:refnum<k34>)
                    n2449 = local read "SET LAB01-1"() -> (w4651:T5)
                    n2450 = local read "DISP LAB01-1"() -> (w4652:T4)
                    n2451 = local read "SIG LAB01-1"() -> (w4656:T2)
                    n2452 = Bundle("FAIL LAB01-1"=w4647, "SIG LAB01-1"=w4656, "TEMP START LAB01-1"=w4655, "DISP LAB01-1"=w4652, "SET LAB01-1"=w4651, "TDMS LAB01-1"=w4654) -> (w4641:T32)  [unwired: 1 in]
                    n2453 = call "sub vi - cycle&temp fail v6.vi"("Amps Lo?"=w4653, "Input Cluster"=w4641, "SELECT"=w4650, "Amps Hi?"=w4649, "Result In"=w4644) -> ("(FAIL) out"=w4646:cluster{"FAIL LO":dbl, "FAIL HI":dbl}, "(DISP) out"=w4642:T4, "T-RISE"=w4643:cluster{"T-RISE (L)":dbl, "T-RISE (N)":dbl}, "Result Out"=w4645:bool, "file error"=w4648:errorcluster)  [unwired: 10 in]
                    n2454 = local write "TEMP RISE LAB01-1"(w4643) -> ()
                    n2455 = local write "FAIL LAB01-1"(w4646) -> ()
                    n2456 = local write "DISP LAB01-1"(w4642) -> ()
                    n2457 = local write "RESULT LAB01-1"(w4645) -> ()
                    n2458 = local write "data file error"(w4648) -> ()
                  }
                }
              }
              frame #1 {
                # "LAB01-2"
                n2459 = case shown="True" w4658 {
                  tunnel: w4660 -> [_ w4673]
                  tunnel: w4657 -> [_ w4670]
                  tunnel: w4659 -> [_ w4669]
                  frame False {
                  }
                  frame True {
                    n2460 = local read "TEMP START LAB01-2"() -> (w4675:cluster{"TL":dbl, "TN":dbl})
                    n2461 = local read "FAIL LAB01-2"() -> (w4666:cluster{"LO":dbl, "HI":dbl})
                    n2462 = local read "TDMS LAB01-2"() -> (w4674:refnum<k34>)
                    n2463 = local read "SET LAB01-2"() -> (w4671:T5)
                    n2464 = local read "DISP LAB01-2"() -> (w4672:T4)
                    n2465 = local read "RESULT LAB01-2"() -> (w4663:bool)
                    n2466 = local read "SIG LAB01-2"() -> (w4676:T2)
                    n2467 = Bundle("FAIL LAB01-2"=w4666, "SIG LAB01-2"=w4676, "TEMP START LAB01-2"=w4675, "DISP LAB01-2"=w4672, "SET LAB01-2"=w4671, "TDMS LAB01-2"=w4674) -> (w4661:T33)  [unwired: 1 in]
                    n2468 = call "sub vi - cycle&temp fail v6.vi"("Amps Lo?"=w4673, "Input Cluster"=w4661, "SELECT"=w4670, "Amps Hi?"=w4669, "Result In"=w4663) -> ("(FAIL) out"=w4665:cluster{"FAIL LO":dbl, "FAIL HI":dbl}, "(DISP) out"=w4668:T4, "T-RISE"=w4662:cluster{"T-RISE (L)":dbl, "T-RISE (N)":dbl}, "Result Out"=w4664:bool, "file error"=w4667:errorcluster)  [unwired: 10 in]
                    n2469 = local write "TEMP RISE LAB01-2"(w4662) -> ()
                    n2470 = local write "FAIL LAB01-2"(w4665) -> ()
                    n2471 = local write "DISP LAB01-2"(w4668) -> ()
                    n2472 = local write "RESULT LAB01-2"(w4664) -> ()
                    n2473 = local write "data file error"(w4667) -> ()
                  }
                }
              }
              frame #2 {
                # "LAB02-1"
                n2474 = case shown="True" w4678 {
                  tunnel: w4680 -> [_ w4693]
                  tunnel: w4677 -> [_ w4690]
                  tunnel: w4679 -> [_ w4689]
                  frame False {
                  }
                  frame True {
                    n2475 = local read "TEMP START LAB02-1"() -> (w4695:cluster{"TL":dbl, "TN":dbl})
                    n2476 = local read "FAIL LAB02-1"() -> (w4686:cluster{"LO":dbl, "HI":dbl})
                    n2477 = local read "TDMS LAB02-1"() -> (w4694:refnum<k34>)
                    n2478 = local read "SET LAB02-1"() -> (w4691:T5)
                    n2479 = local read "DISP LAB02-1"() -> (w4692:T4)
                    n2480 = local read "SIG LAB02-1"() -> (w4696:T2)
                    n2481 = local read "RESULT LAB02-1"() -> (w4683:bool)
                    n2482 = Bundle("FAIL LAB02-1"=w4686, "SIG LAB02-1"=w4696, "TEMP START LAB02-1"=w4695, "DISP LAB02-1"=w4692, "SET LAB02-1"=w4691, "TDMS LAB02-1"=w4694) -> (w4681:T34)  [unwired: 1 in]
                    n2483 = call "sub vi - cycle&temp fail v6.vi"("Amps Lo?"=w4693, "Input Cluster"=w4681, "SELECT"=w4690, "Amps Hi?"=w4689, "Result In"=w4683) -> ("(FAIL) out"=w4685:cluster{"FAIL LO":dbl, "FAIL HI":dbl}, "(DISP) out"=w4688:T4, "T-RISE"=w4682:cluster{"T-RISE (L)":dbl, "T-RISE (N)":dbl}, "Result Out"=w4684:bool, "file error"=w4687:errorcluster)  [unwired: 10 in]
                    n2484 = local write "TEMP RISE LAB02-1"(w4682) -> ()
                    n2485 = local write "FAIL LAB02-1"(w4685) -> ()
                    n2486 = local write "DISP LAB02-1"(w4688) -> ()
                    n2487 = local write "RESULT LAB02-1"(w4684) -> ()
                    n2488 = local write "data file error"(w4687) -> ()
                  }
                }
              }
              frame #3 {
                # "LAB02-2"
                n2489 = case shown="True" w4698 {
                  tunnel: w4700 -> [_ w4713]
                  tunnel: w4697 -> [_ w4710]
                  tunnel: w4699 -> [_ w4709]
                  frame False {
                  }
                  frame True {
                    n2490 = local read "TEMP START LAB02-2"() -> (w4715:cluster{"TL":dbl, "TN":dbl})
                    n2491 = local read "FAIL LAB02-2"() -> (w4706:cluster{"LO":dbl, "HI":dbl})
                    n2492 = local read "TDMS LAB02-2"() -> (w4714:refnum<k34>)
                    n2493 = local read "SET LAB02-2"() -> (w4711:T5)
                    n2494 = local read "DISP LAB02-2"() -> (w4712:T4)
                    n2495 = local read "SIG LAB02-2"() -> (w4716:T2)
                    n2496 = local read "RESULT LAB02-2"() -> (w4703:bool)
                    n2497 = Bundle("FAIL LAB02-2"=w4706, "SIG LAB02-2"=w4716, "TEMP START LAB02-2"=w4715, "DISP LAB02-2"=w4712, "SET LAB02-2"=w4711, "TDMS LAB02-2"=w4714) -> (w4701:T35)  [unwired: 1 in]
                    n2498 = call "sub vi - cycle&temp fail v6.vi"("Amps Lo?"=w4713, "Input Cluster"=w4701, "SELECT"=w4710, "Amps Hi?"=w4709, "Result In"=w4703) -> ("(FAIL) out"=w4705:cluster{"FAIL LO":dbl, "FAIL HI":dbl}, "(DISP) out"=w4708:T4, "T-RISE"=w4702:cluster{"T-RISE (L)":dbl, "T-RISE (N)":dbl}, "Result Out"=w4704:bool, "file error"=w4707:errorcluster)  [unwired: 10 in]
                    n2499 = local write "TEMP RISE LAB02-2"(w4702) -> ()
                    n2500 = local write "FAIL LAB02-2"(w4705) -> ()
                    n2501 = local write "DISP LAB02-2"(w4708) -> ()
                    n2502 = local write "RESULT LAB02-2"(w4704) -> ()
                    n2503 = local write "data file error"(w4707) -> ()
                  }
                }
              }
              frame #4 {
                # "LAB03-1"
                n2504 = case shown="True" w4718 {
                  tunnel: w4720 -> [_ w4733]
                  tunnel: w4717 -> [_ w4730]
                  tunnel: w4719 -> [_ w4729]
                  frame False {
                  }
                  frame True {
                    n2505 = local read "TEMP START LAB03-1"() -> (w4735:cluster{"TL":dbl, "TN":dbl})
                    n2506 = local read "FAIL LAB03-1"() -> (w4726:cluster{"LO":dbl, "HI":dbl})
                    n2507 = local read "TDMS LAB03-1"() -> (w4734:refnum<k34>)
                    n2508 = local read "SET LAB03-1"() -> (w4731:T5)
                    n2509 = local read "DISP LAB03-1"() -> (w4732:T4)
                    n2510 = local read "SIG LAB03-1"() -> (w4736:T2)
                    n2511 = local read "RESULT LAB03-1"() -> (w4723:bool)
                    n2512 = Bundle("FAIL LAB03-1"=w4726, "SIG LAB03-1"=w4736, "TEMP START LAB03-1"=w4735, "DISP LAB03-1"=w4732, "SET LAB03-1"=w4731, "TDMS LAB03-1"=w4734) -> (w4721:T36)  [unwired: 1 in]
                    n2513 = call "sub vi - cycle&temp fail v6.vi"("Amps Lo?"=w4733, "Input Cluster"=w4721, "SELECT"=w4730, "Amps Hi?"=w4729, "Result In"=w4723) -> ("(FAIL) out"=w4725:cluster{"FAIL LO":dbl, "FAIL HI":dbl}, "(DISP) out"=w4728:T4, "T-RISE"=w4722:cluster{"T-RISE (L)":dbl, "T-RISE (N)":dbl}, "Result Out"=w4724:bool, "file error"=w4727:errorcluster)  [unwired: 10 in]
                    n2514 = local write "TEMP RISE LAB03-1"(w4722) -> ()
                    n2515 = local write "FAIL LAB03-1"(w4725) -> ()
                    n2516 = local write "DISP LAB03-1"(w4728) -> ()
                    n2517 = local write "RESULT LAB03-1"(w4724) -> ()
                    n2518 = local write "data file error"(w4727) -> ()
                  }
                }
              }
              frame #5 {
                # "LAB03-2"
                n2519 = case shown="True" w4738 {
                  tunnel: w4740 -> [_ w4753]
                  tunnel: w4737 -> [_ w4750]
                  tunnel: w4739 -> [_ w4749]
                  frame False {
                  }
                  frame True {
                    n2520 = local read "TEMP START LAB03-2"() -> (w4755:cluster{"TL":dbl, "TN":dbl})
                    n2521 = local read "FAIL LAB03-2"() -> (w4746:cluster{"LO":dbl, "HI":dbl})
                    n2522 = local read "TDMS LAB03-2"() -> (w4754:refnum<k34>)
                    n2523 = local read "SET LAB03-2"() -> (w4751:T5)
                    n2524 = local read "DISP LAB03-2"() -> (w4752:T4)
                    n2525 = local read "RESULT LAB03-2"() -> (w4743:bool)
                    n2526 = local read "SIG LAB03-2"() -> (w4756:T2)
                    n2527 = Bundle("FAIL LAB03-2"=w4746, "SIG LAB03-2"=w4756, "TEMP START LAB03-2"=w4755, "DISP LAB03-2"=w4752, "SET LAB03-2"=w4751, "TDMS LAB03-2"=w4754) -> (w4741:T37)  [unwired: 1 in]
